vi "Check Invok Node Error.vi"(3 "Connect":i32, 4 "error in (no error)":errorcluster, 5 "MC switch refnum in":refnum<k24>) -> (1 "error out":errorcluster, 2 "MC switch refnum out":refnum<k24>)   [LabVIEW 2019, in "Minicircuit RF Switch Box.lvlib"]
uses:
  <instrlib>/LV_Minicircuit_RF_Switch/Minicircuit RF Switch Box.lvlib
  C:/Program Files (x86)/National Instruments/LabVIEW 2019/instr.lib/LV_Minicircuit_RF_Switch/mcl_RF_Switch_Controller_NET45.dll
  mcl_RF_Switch_Controller_NET45.dll
  <vilib>/Utility/error.llb/Error Cluster From Error Code.vi
  <vilib>/ErrorRing/Error Ring.xnode
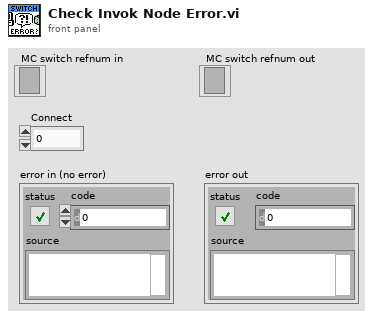
[diagram p1: front panel]
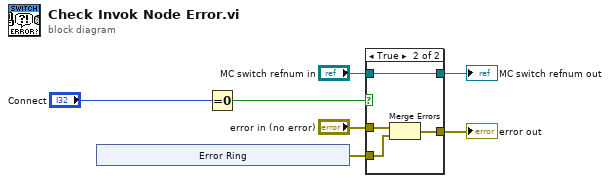
[diagram p0: block diagram]
diagram:
  n1 = xnode "Error Ring"() -> ("error out"=w5:errorcluster)
  n2 = Equal To 0?(x="Connect") -> (x = 0?=w2:bool)
  n3 = case shown="True" w2 {
    tunnel: "error in (no error)" -> [w9 w13]
    tunnel: [w9 w12] -> w7
    tunnel: [w8 w11] -> w6
    tunnel: "MC switch refnum in" -> [w8 w11]
    tunnel: w5 -> [_ w10]
    frame False {
    }
    frame True {
      n4 = Merge Errors(w13, w10) -> (w12:errorcluster)
    }
  }
  "error out" <- w7
  "MC switch refnum out" <- w6
